vi "Datasavetemplate.vi"() -> ()   [LabVIEW 2021]
uses:
  <vilib>/Utility/file.llb/Write Delimited Spreadsheet (DBL).vi
panel:
  out "loop count":i32
  in  "file path (dialog if empty)":path
  out "Waveform Chart":dbl(graph)
  out "Loop measurement":dbl
  out "Array":dbl[](array[numeric])
  in  "Record":bool
  out "Live measurement":dbl
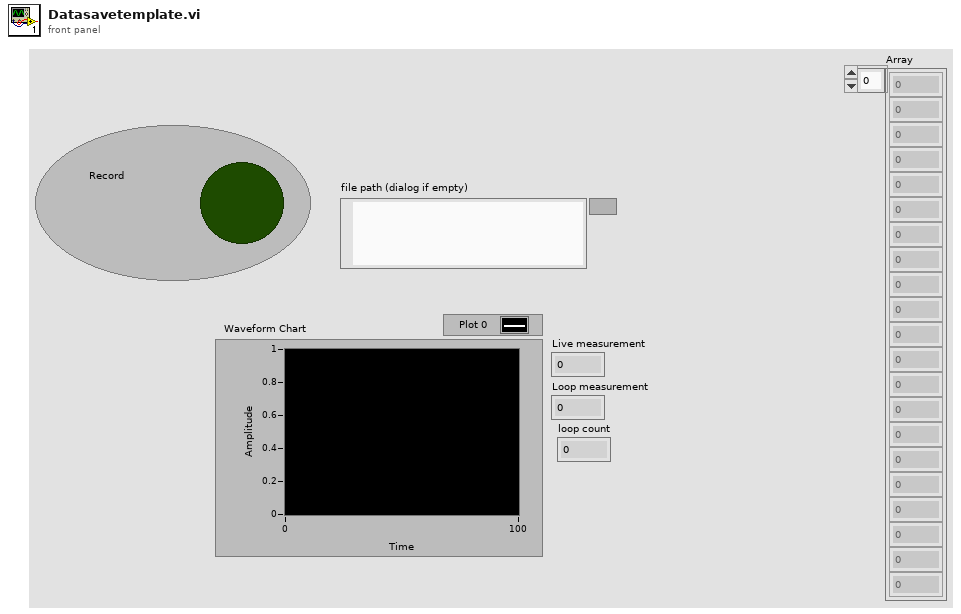
[diagram p1: front panel]
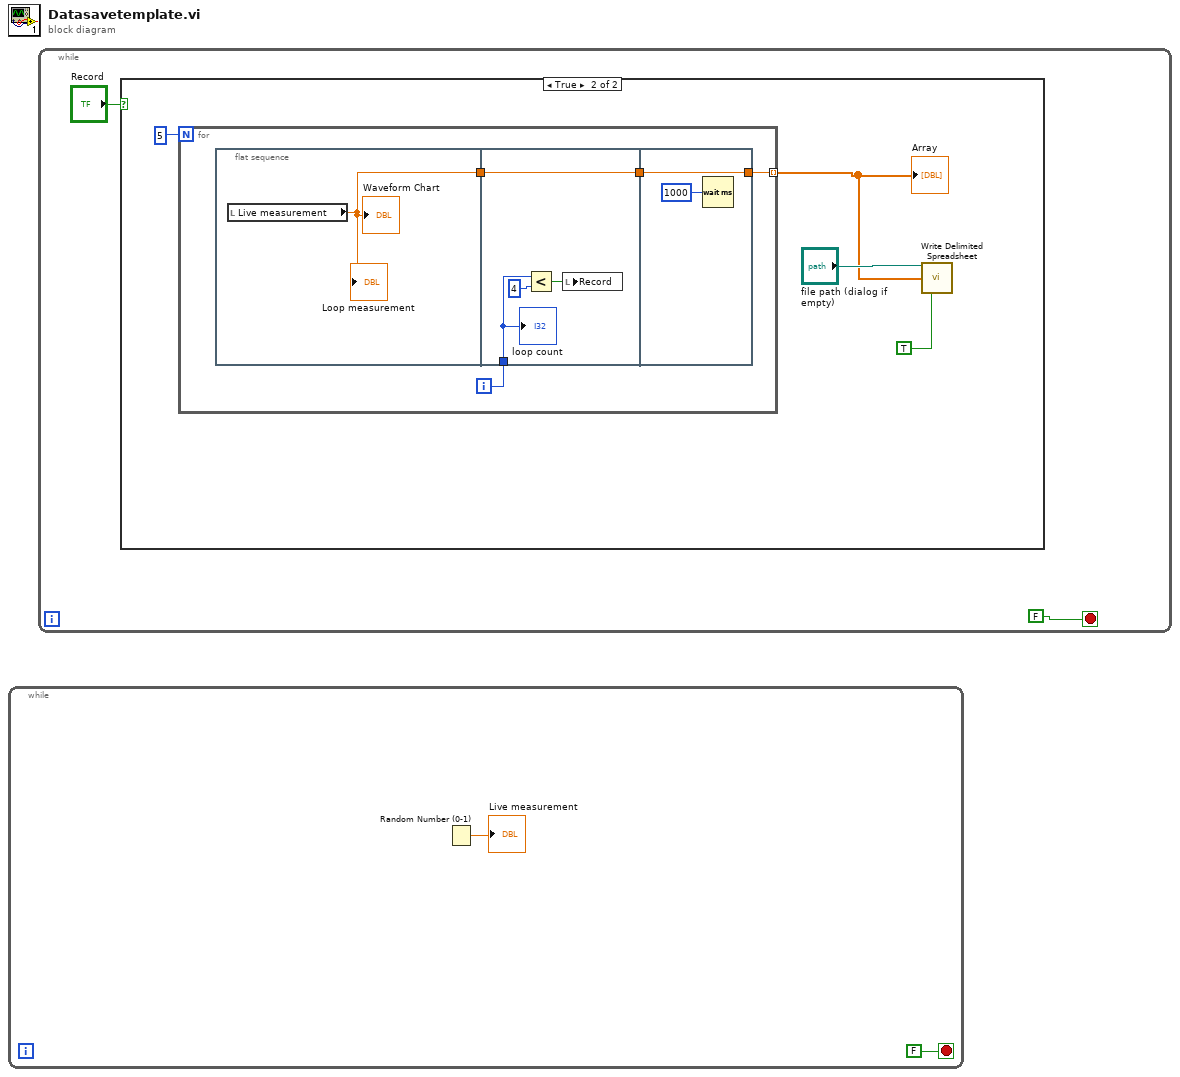
[diagram p0: block diagram]
diagram:
  n1 = while {
    stop <- FALSE stop-if-true
    n2 = Random Number (0-1)() -> (number: 0 to 1=→"Live measurement":dbl)
  }
  n3 = while {
    stop <- FALSE stop-if-true
    n4 = case shown="True" "Record" {
      frame False {
        # "do nothing"
      }
      frame True {
        n5 = for {
          N: 5 -> [_]
          tunnel: [w12] -> w6 mode=indexing
          i -> [w10]
          n6 = flat-sequence {
            tunnel: [w13] -> w11
            tunnel: w11 -> [w17]
            tunnel: w10 -> [w14]
            tunnel: [w17] -> w9
            tunnel: [w19] -> w12
            tunnel: w9 -> [w19]
            frame #0 {
              n7 = local read "Live measurement"() -> (w13:dbl)
              "Loop measurement" <- w13
              "Waveform Chart" <- w13
            }
            frame #1 {
              n8 = Less?(x=w14, y=4) -> (x < y?=w16:bool)
              n9 = local write "Record"(w16) -> ()
              "loop count" <- w14
            }
            frame #2 {
              n10 = Wait (ms)(milliseconds to wait=u32 1000) -> ()  [unwired: 1 out]
            }
          }
        }
        "Array" <- w6
        n11 = call-poly <vilib>:"Write Delimited Spreadsheet.vi"("file path (dialog if empty)"="file path (dialog if empty)", "1D data"=w6, "transpose? (no:F)"=TRUE) -> ()  [unwired: 11 in, 2 out]
      }
    }
  }
